vi "Read Configuration File.vi"(8 "error in (no error)":errorcluster, 11 "Example Instrument in":refnum<class "Instrument.LN2.lvclass">) -> (0 "error out":errorcluster, 3 "LN2":refnum<class "Instrument.LN2.lvclass">)   [LabVIEW 2019, in "Instrument.LN2.lvclass"]
uses:
  Instrument.LN2.lvclass
  <userlib>/LevyLab/Instrument Framework/Instrument Types/VSource/Instrument.VSource.lvclass
  <userlib>/LevyLab/Instrument Framework/SMOs/Instrument/Instrument.lvclass
  <userlib>/LevyLab/Instrument Framework/SMOs/Configuration/Configuration.lvclass
  C:/Program Files (x86)/National Instruments/LabVIEW 2019/user.lib/LevyLab/Instrument Framework/SMOs/Instrument/Instrument.lvclass
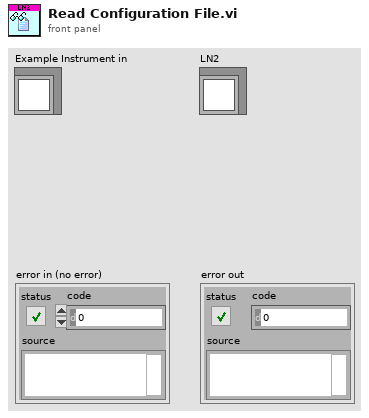
[diagram p1: front panel]
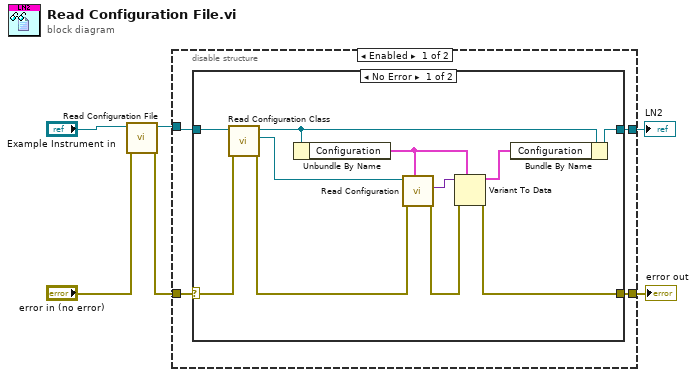
[diagram p0: block diagram]
diagram:
  n1 = call-parent "Read Configuration File.vi"("error in (no error)"="error in (no error)", "Instrument in"="Example Instrument in") -> ("error out"=w2:errorcluster, "Instrument out"=w1:refnum<class "Instrument.LN2.lvclass">)  [unwired: 8 in]
  n2 = disable-structure shown="Enabled" {
    disable-tunnel: [w10 w25] -> w6
    disable-tunnel: [w9 w24] -> w5
    disable-tunnel: w2 -> [w8 w24]
    disable-tunnel: w1 -> [w7 w25]
    frame Enabled {
      n3 = case shown="No Error" w8 {
        selector: w8 -> [w17 w23]
        tunnel: w7 -> [w19 w22]
        tunnel: [w15 w22] -> w10
        tunnel: [w18 w23] -> w9
        frame No Error {
          n4 = call <userlib>:"Read Configuration Class.vi"("error in (no error)"=w17, "Instrument in"=w19) -> ("error out"=w20:errorcluster, "Configuration"=w11:refnum<class "Configuration.lvclass">, "Instrument out"=w14:refnum<class "Instrument.LN2.lvclass">)  [unwired: 7 in]
          n5 = Unbundle By Name(w14) -> ("Configuration"=w16:cluster{"Fridge":string})
          n6 = call <userlib>:"Read Configuration.vi"("INI Fomatted Cluster Type"=w16, "error in (no error)"=w20, "Configuration in"=w11) -> ("error out"=w21:errorcluster, "Configuration"=w13:variant)  [unwired: 6 in, 1 out]
          n7 = Variant To Data(error in=w21, type=w16, Variant=w13) -> (data=w12:cluster{"Fridge":string}, error out=w18:errorcluster)
          n8 = Bundle By Name(cluster=w14, "Configuration"=w12) -> (w15:refnum<class "Instrument.LN2.lvclass">)
        }
        frame Error {
        }
      }
    }
    frame Disabled {
    }
  }
  "LN2" <- w6
  "error out" <- w5
